vi "CT_SetPWMLevel.vi"(8 "error in (no error)":errorcluster, 9 "PWM Frequency":dbl, 10 "Duty Cycle %":dbl, 11 "Task In":refnum<k21>) -> (0 "error out":errorcluster, 3 "Task Out":refnum<k21>)   [LabVIEW 2009]
uses:
  Program Files (x86)/National Instruments/LabVIEW 2009/resource/objmgr/daqmx.rc
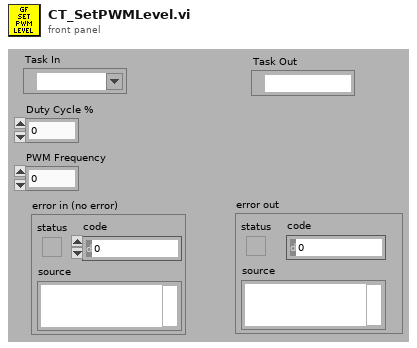
[diagram p1: front panel]
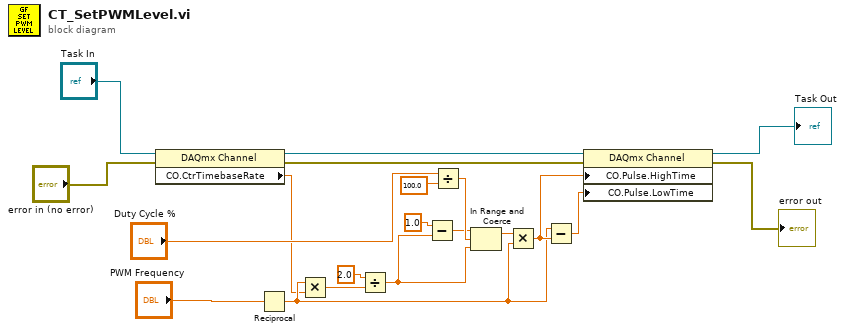
[diagram p0: block diagram]
diagram:
  n1 = property class="DAQmx Channel"(reference="Task In", error in="error in (no error)") -> (reference out=w16:refnum<k21>, error out=w15:errorcluster, "CO.CtrTimebaseRate"=w13:dbl)
  n2 = Reciprocal(x="PWM Frequency") -> (1/x=w14:dbl)
  n3 = Multiply(x=w14, y=w13) -> (x*y=w12:dbl)
  n4 = Divide(x=2.0, y=w12) -> (x/y=w6:dbl)
  n5 = Subtract(x=1.0, y=w6) -> (x-y=w7:dbl)
  n6 = Divide(x="Duty Cycle %", y=100.0) -> (x/y=w10:dbl)
  n7 = In Range and Coerce(upper limit=w7, x=w10, lower limit=w6) -> (coerced(x)=w9:dbl)  [unwired: 1 out]
  n8 = Multiply(x=w9, y=w14) -> (x*y=w18:dbl)
  n9 = Subtract(x=w14, y=w18) -> (x-y=w17:dbl)
  n10 = property class="DAQmx Channel"(reference=w16, error in=w15, "CO.Pulse.HighTime"=w18, "CO.Pulse.LowTime"=w17) -> (reference out=→"Task Out":refnum<k21>, error out=→"error out":errorcluster)
